vi "dbg.auth.vi"() -> ()   [LabVIEW 2015, in "DDC_7976R_v1.lvlib"]
uses:
  DDC_7976R_v1.lvlib
panel:
  in  "rnd.U64":u32
  out "dbg.auth.en":bool
  in  "dbg.auth.pass":u64
  out "dbg.lic.error":bool
  in  "dbg.auth.code":u64
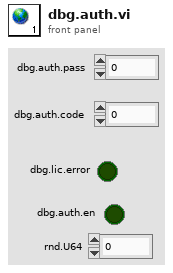
[diagram p1: front panel]
diagram:
